vi "WLAN_SigContent.vi"(8 "error in (no error)":errorcluster, 10 "Frequency channel estimation":cdb[](array[numeric]) format="%.6g", 11 "SIG":cdb[](array[numeric])) -> (0 "error out":errorcluster, 1 "Symbol numbers":i32, 2 "encoded bit numbers":u32, 3 "original bit numbers":u32, 4 "Modulation parameter":T1, 5 "SIG valid?":bool)   [LabVIEW 2018]
panel:
  out "size(s) 2":i32
  out "size(s)":i32
  out "output bit stream":i8[](array[numeric])
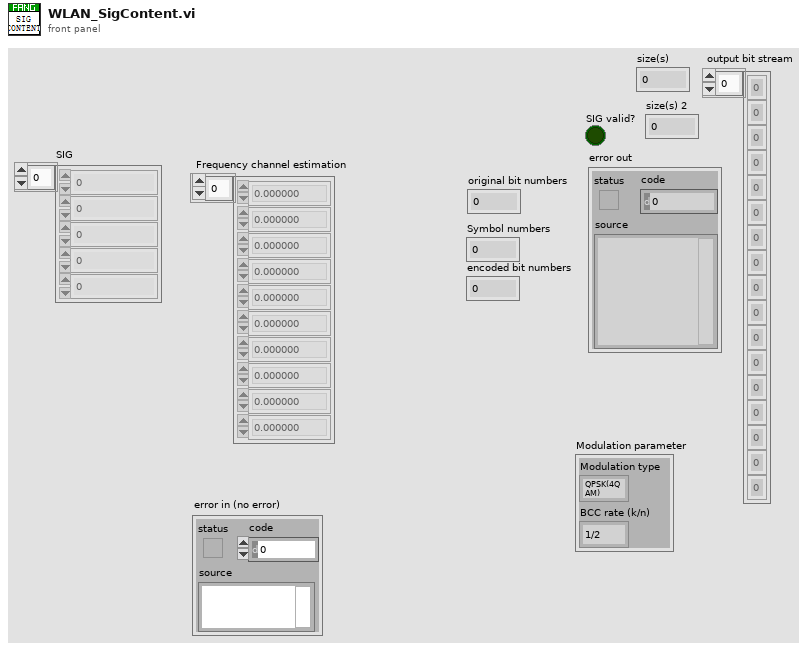
[diagram p1: front panel]
types:
  T1 = cluster{"Modulation type":enum16{"QPSK(4QAM)", "64QAM", "16QAM", "BPSK"}, "BCC rate (k/n)":enum16{"1/2", "2/3", "3/4"}}
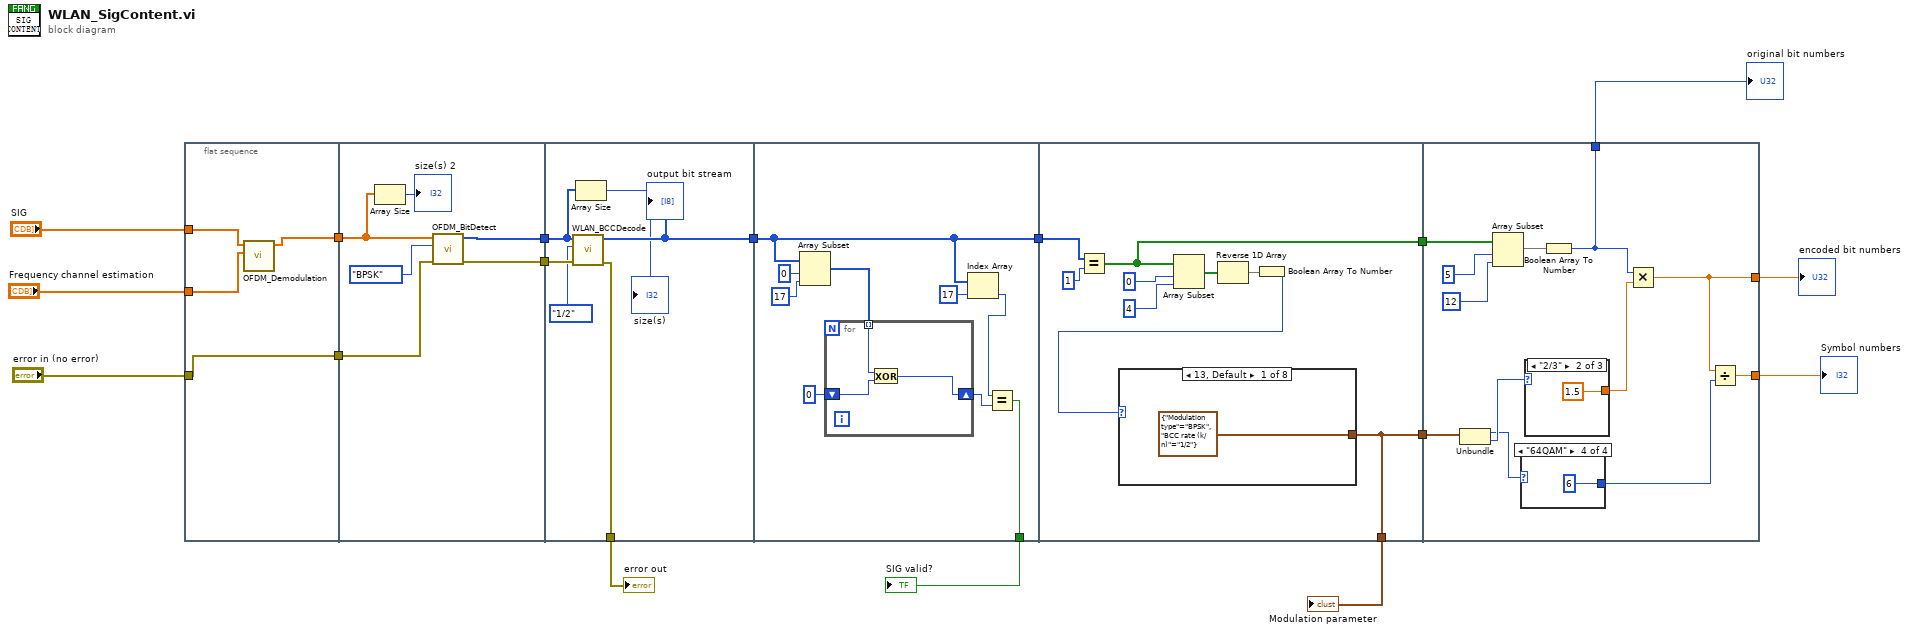
[diagram p0: block diagram]
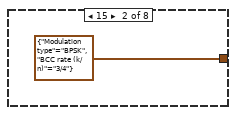
[diagram p2: hidden frame]
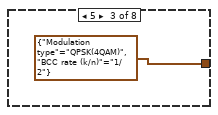
[diagram p3: hidden frame]
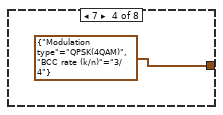
[diagram p4: hidden frame]
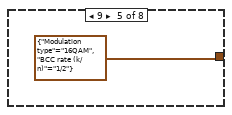
[diagram p5: hidden frame]
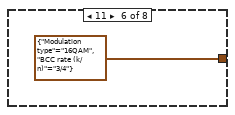
[diagram p6: hidden frame]
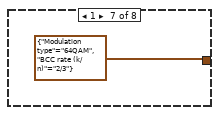
[diagram p7: hidden frame]
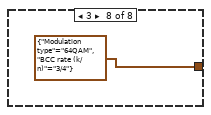
[diagram p8: hidden frame]
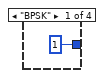
[diagram p9: hidden frame]
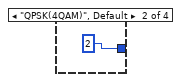
[diagram p10: hidden frame]
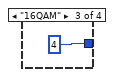
[diagram p11: hidden frame]
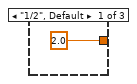
[diagram p12: hidden frame]
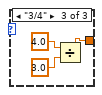
[diagram p13: hidden frame]
diagram:
  n1 = flat-sequence {
    tunnel: [w21] -> w17
    tunnel: "SIG" -> [w20]
    tunnel: "Frequency channel estimation" -> [w19]
    tunnel: [w18] -> w11
    tunnel: "error in (no error)" -> [w18]
    tunnel: w17 -> [w24]
    tunnel: [w27] -> w14
    tunnel: [w26] -> w12
    tunnel: w11 -> [w25]
    tunnel: w14 -> [w30]
    tunnel: [w33] -> w7
    tunnel: w12 -> [w32]
    tunnel: [w31] -> w2
    tunnel: w7 -> [w39]
    tunnel: [w39] -> w6
    tunnel: [w35] -> w1
    tunnel: w6 -> [w53]
    tunnel: [w50] -> w13
    tunnel: [w46] -> w5
    tunnel: [w46] -> w4
    tunnel: w13 -> [w72]
    tunnel: [w69] -> w9
    tunnel: [w70] -> w8
    tunnel: w4 -> [w68]
    tunnel: [w63] -> w3
    frame #0 {
      n2 = call "OFDM_Demodulation.vi"("Frequency channel estimation"=w19, "Input sequence"=w20) -> ("Output sequence"=w21:cdb[])  [unwired: 9 in]
    }
    frame #1 {
      n3 = Array Size(array=w24) -> (size(s)=→"size(s) 2":i32)
      n4 = call "OFDM_BitDetect.vi"("Input symbols"=w24, "Modulation type"=enum16{"QPSK(4QAM)", "64QAM", "16QAM", "BPSK"}."BPSK", "error in (no error)"=w25) -> ("Output bits"=w27:i8[], "error out"=w26:errorcluster)  [unwired: 6 in]
    }
    frame #2 {
      n5 = call "WLAN_BCCDecode.vi"("error in (no error)"=w32, "BCC rate (k/n)"=enum16{"1/2", "2/3", "3/4"}."1/2", "input bit stream"=w30) -> ("error out"=w31:errorcluster, "output bit stream"=w33:i8[])  [unwired: 7 in]
      "output bit stream" <- w33
      n6 = Array Size(array=w30) -> (size(s)=→"size(s)":i32)
    }
    frame #3 {
      n7 = Array Subset(array=w39, index=0, length=17) -> (w41:i8[])
      n8 = for {
        shift-right: [w44] -> w36
        shift-left: i8 0 -> [w45]
        tunnel: w41 -> [w43] mode=indexing
        n9 = Exclusive Or(1:w45, 2:w43) -> (0:w44:i8)
      }
      n10 = Index Array(array=w39, index=17) -> (element=w37:i8)
      n11 = Equal?(x=w37, y=w36) -> (x = y?=w35:bool)
    }
    frame #4 {
      n12 = Equal?(x=w53, y=1 ("length")) -> (x = y?=w50:bool[])
      n13 = Array Subset(array=w50, index=0, length=4) -> (w49:bool[])
      n14 = Reverse 1D Array(array=w49) -> (reversed array=w48:bool[])
      n15 = Boolean Array To Number(Boolean array=w48) -> (number=w47:u32)
      n16 = case shown="13, Default" w47 {
        tunnel: [T1 {"Modulation type"=enum."BPSK", "BCC rate (k/n)"=enum."1/2"} ("Modulation parameter") T1 {"Modulation type"=enum."BPSK", "BCC rate (k/n)"=enum."3/4"} ("Modulation parameter") T1 {"Modulation type"=enum."QPSK(4QAM)", "BCC rate (k/n)"=enum."1/2"} ("Modulation parameter") T1 {"Modulation type"=enum."QPSK(4QAM)", "BCC rate (k/n)"=enum."3/4"} ("Modulation parameter") T1 {"Modulation type"=enum."16QAM", "BCC rate (k/n)"=enum."1/2"} ("Modulation parameter") T1 {"Modulation type"=enum."16QAM", "BCC rate (k/n)"=enum."3/4"} ("Modulation parameter") T1 {"Modulation type"=enum."64QAM", "BCC rate (k/n)"=enum."2/3"} ("Modulation parameter") T1 {"Modulation type"=enum."64QAM", "BCC rate (k/n)"=enum."3/4"} ("Modulation parameter")] -> w46
        frame 13, Default {
        }
        frame 15 {
        }
        frame 5 {
        }
        frame 7 {
        }
        frame 9 {
        }
        frame 11 {
        }
        frame 1 {
        }
        frame 3 {
        }
      }
    }
    frame #5 {
      n17 = Unbundle(w68) -> ("Modulation type"=w66:enum16{"QPSK(4QAM)", "64QAM", "16QAM", "BPSK"}, "BCC rate (k/n)"=w67:enum16{"1/2", "2/3", "3/4"})
      n18 = Array Subset(array=w72, index=5, length=12) -> (w71:bool[])
      n19 = case shown="\"64QAM\"" w66 {
        tunnel: [1 2 4 6] -> w64
        frame "BPSK" {
        }
        frame "QPSK(4QAM)", Default {
        }
        frame "16QAM" {
        }
        frame "64QAM" {
        }
      }
      n20 = case shown="\"2/3\"" w67 {
        tunnel: [2.0 1.5 w83] -> w65
        frame "1/2", Default {
        }
        frame "2/3" {
        }
        frame "3/4" {
          n21 = Divide(x=4.0, y=3.0) -> (x/y=w83:dbl)
        }
      }
      n22 = Boolean Array To Number(Boolean array=w71) -> (number=w69:u32)
      n23 = Multiply(x=w69, y=w65) -> (x*y=w63:dbl)
      n24 = Divide(x=w63, y=w64) -> (x/y=w70:dbl)
    }
  }
  "original bit numbers" <- w9
  "Symbol numbers" <- w8
  "Modulation parameter" <- w5
  "encoded bit numbers" <- w3
  "error out" <- w2
  "SIG valid?" <- w1
